vi "禹山溶解氧_获取温度和测量值.vi"(5 "大气压补偿":dbl=1.0, 7 "盐度补偿":dbl, 8 "error in (no error)":errorcluster caption="错误输入（无错误）", 11 "MB session in":refnum<class "MB_Master.lvclass">) -> (0 "error out":errorcluster caption="错误输出", 2 "输出值":cluster{"温度测量值":sgl, "DO%":sgl, "DOmg/L":sgl}, 3 "MB session out":refnum<class "MB_Master.lvclass">)   [LabVIEW 2016, in "斯坦道多参数.lvlib"]
uses:
  <vilib>/Plasmionique/MB Master/MB_Master/MB_Master.lvclass
  <vilib>/Plasmionique/MB Master/MB Master.lvlib
  <vilib>/ptbypt/NI_PtbyPt.lvlib
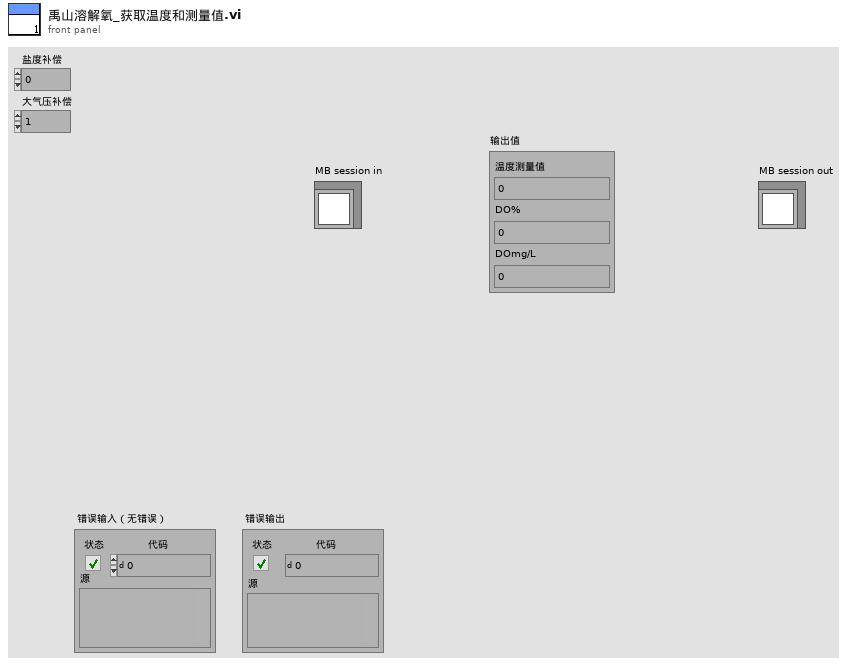
[diagram p1: front panel]
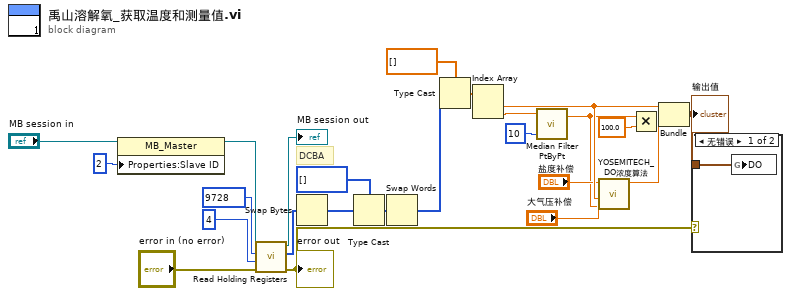
[diagram p0: block diagram]
diagram:
  # "DCBA"
  n1 = property class="MB_Master"(reference="MB session in", "Properties:Slave ID"=u16 2 ("y")) -> (reference out=w17:refnum<class "MB_Master.lvclass">)  [unwired: 1 in, 1 out]
  n2 = call <vilib>:"Read Holding Registers.vi"("error in (no error)"="error in (no error)", "quantity"=u16 4, "starting address"=u16 9728, "MB session in"=w17) -> ("error out"=w7:errorcluster, "Registers"=w15:u16[], "MB session out"=→"MB session out":refnum<class "MB_Master.lvclass">)  [unwired: 5 in]
  "error out" <- w7
  n3 = Swap Bytes(anything=w15) -> (byte swapped=w14:u16[])
  n4 = Type Cast(type=u32[] [] ("数组 2"), x=w14) -> (*(type *) &x=w21:u32[])
  n5 = Swap Words(1:w21) -> (0:w23:u32[])
  n6 = Type Cast(type=sgl[] [] ("数组 2"), x=w23) -> (*(type *) &x=w19:sgl[])
  n7 = Index Array(array=w19) -> (element #1=w13:sgl, element #2=w2:sgl)  [unwired: 2 in]
  n8 = call <vilib>:"Median Filter PtByPt.vi"("rank"=10, "x"=w2) -> ("Filtered x"=w1:dbl)  [unwired: 2 in, 1 out]
  n9 = call "YOSEMITECH_DO浓度算法.vi"("溶解氧饱和度值"=w1, "水温"=w13, "大气压补偿"="大气压补偿", "盐度补偿"="盐度补偿") -> ("DataDo_mgL"=w12:dbl)  [unwired: 7 in]
  n10 = Multiply(x=w1, y=sgl 100.0) -> (x*y=w9:dbl)
  n11 = Bundle("数值"=w13, w9, "DataDo_mgL"=w12) -> (w6:cluster{"数值":sgl, dbl, "DataDo_mgL":dbl})  [unwired: 1 in]
  "输出值" <- w6
  n12 = case shown="无错误" w7 {
    tunnel: w6 -> [w26 _]
    frame No Error {
      n13 = global write "禹山过程全局变量.vi" "DO"(w26) -> ()
    }
    frame Error {
    }
  }
